vi "QMH_Create_User_Event.vi"(8 "error in (no error)":errorcluster caption="entrée d'erreur (pas d'erreur)") -> (0 "error out":errorcluster caption="sortie d'erreur", 2 "User Stop Event":refnum<user-event>, 3 "Refnum register for events":refnum<event-registration>)   [LabVIEW 2015]
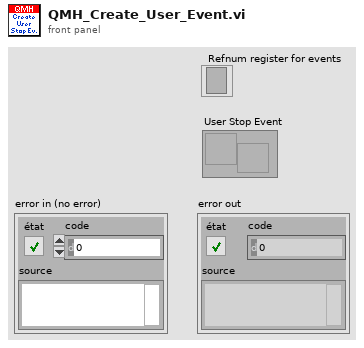
[diagram p1: front panel]
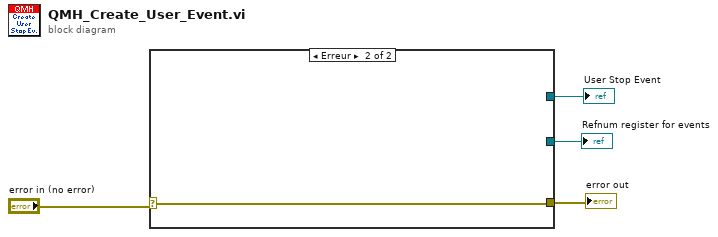
[diagram p0: block diagram]
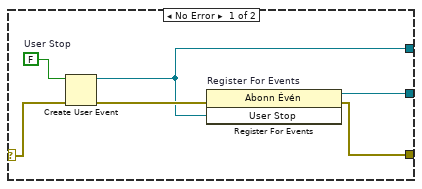
[diagram p2: hidden frame]
diagram:
  n1 = case shown="Erreur" "error in (no error)" {
    selector: "error in (no error)" -> [w6 w11]
    tunnel: [w10 _] -> w4
    tunnel: [w7 _] -> w3
    tunnel: [w5 w11] -> w1
    frame No Error {
      w8 = FALSE  # User Stop
      n2 = Create User Event(user event datatype=w8, error in=w6) -> (user event=w7:refnum<user-event>, error out=w9:errorcluster)
      n3 = register-events "Register For Events"(error in=w9, w7) -> (reference out=w10:refnum<event-registration>, error out=w5:errorcluster)  [unwired: 1 in]
    }
    frame Error {
    }
  }
  "Refnum register for events" <- w4
  "User Stop Event" <- w3
  "error out" <- w1
